vi "SyntaxToken.vi"(8 "error in":errorcluster, 9 "Error Index In":i32, 10 "Funcion Analizada":string, 11 "Logical Parsed Expression":T1) -> (0 "error out":errorcluster, 1 "Error Index Out":i32, 2 "Token":string[](array[string]), 3 "Logical Parsed Expression Out":T1)   [LabVIEW 2014]
uses:
  TypeDefs/LogicParsedExpression.ctl
  <vilib>/regexp/Match Regular Expression.xnode
  SeqLoop.lvlib
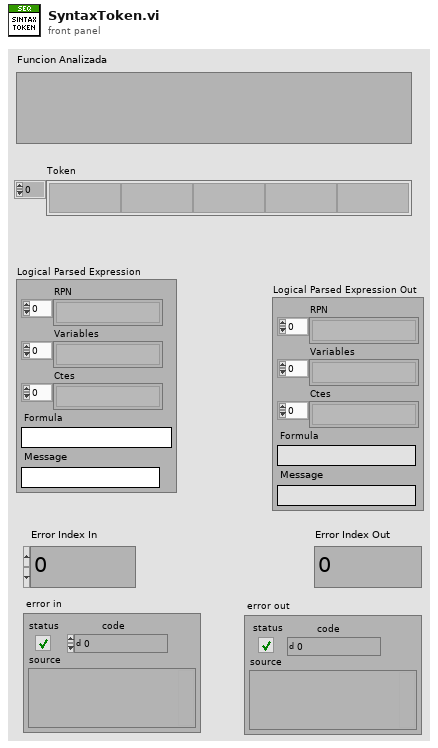
[diagram p1: front panel]
types:
  T1 = typedef "SeqLoop.lvlib/LogicParsedExpression.ctl" = cluster{"RPN ":string[], "Variables":string[], "Ctes":string[], "Formula":string, "Message":string}
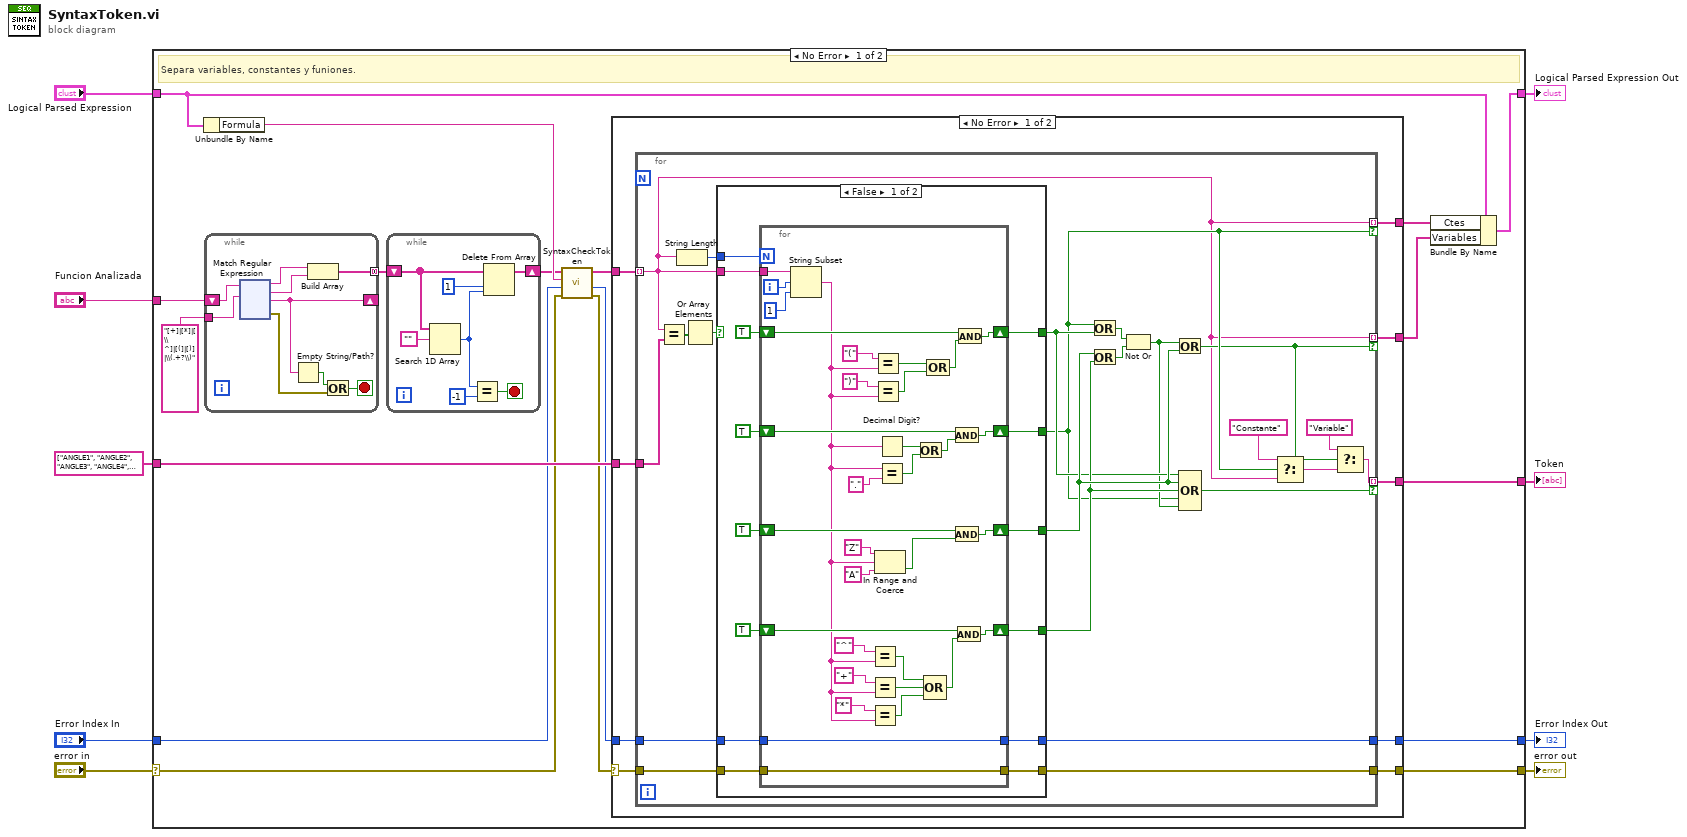
[diagram p0: block diagram]
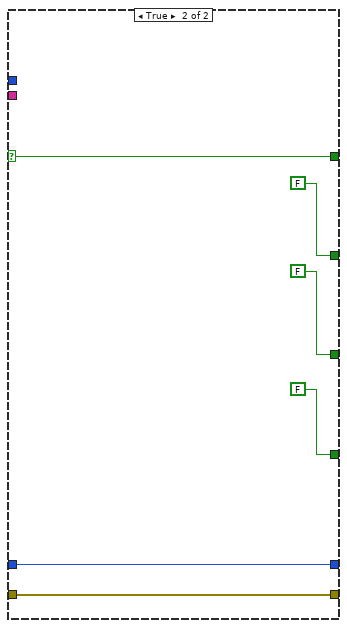
[diagram p2: hidden frame]
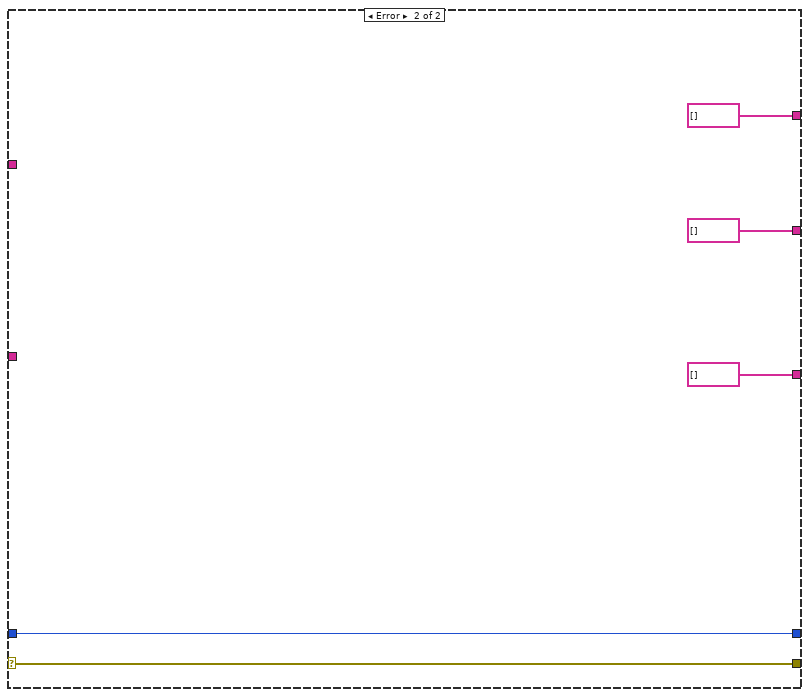
[diagram p3: hidden frame]
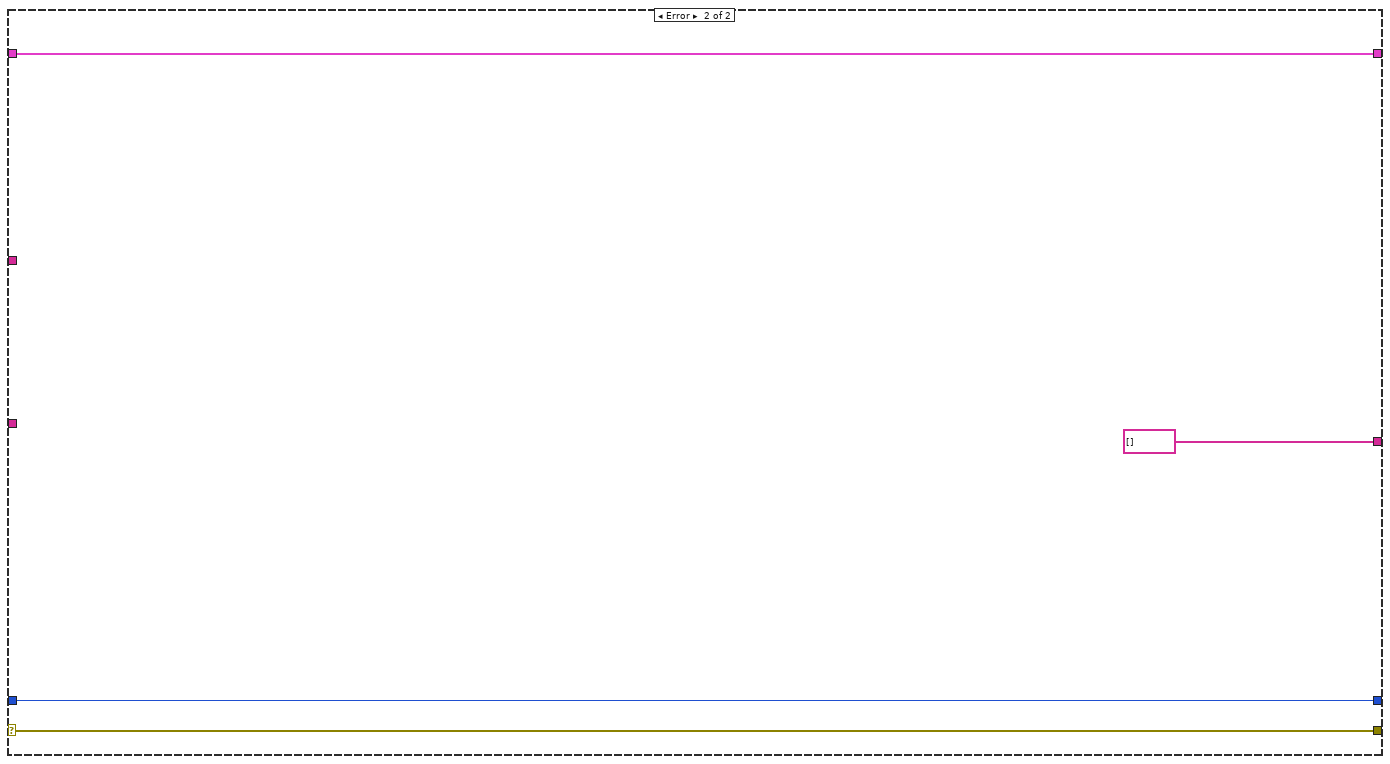
[diagram p4: hidden frame]
diagram:
  n1 = case shown="No Error" "error in" {
    selector: "error in" -> [w13 w250]
    tunnel: [w23 w250] -> w8
    tunnel: [w24 w249] -> w2
    tunnel: "Logical Parsed Expression" -> [w20 w249]
    tunnel: string[] ["ANGLE1", "ANGLE2", "ANGLE3", "ANGLE4", "ANGLE5", "NO", "W"] ("Funciones") -> [w22 _]
    tunnel: [w21 string[] []] -> w7
    tunnel: "Funcion Analizada" -> [w19 _]
    tunnel: "Error Index In" -> [w12 w247]
    tunnel: [w18 w247] -> w4
    frame No Error {
      # "Separa variables, constantes y funiones."
      n2 = Unbundle By Name(w20) -> ("Formula"=w11:string)
      n3 = while {
        tunnel: "[+]|[*]|[\\^]|[(]|[)]|\\(.+?\\)" ("regular expression") -> [w131]
        shift-right: [w130] -> _
        shift-left: w19 -> [w132]
        tunnel: [w129] -> w26 mode=concatenating
        stop <- w125 stop-if-true
        n4 = xnode "Match Regular Expression"("input string"=w132, "regular expression"=w131) -> ("before match"=w128:string, "whole match"=w127:string, "after match"=w130:string, "error out"=w124:errorcluster)  [unwired: 4 in, 1 out]
        n5 = Empty String/Path?(string/path=w130) -> (empty?=w126:bool)
        n6 = Build Array(w128, w127) -> (w129:string[])
        n7 = Or(x=w126, y=w124) -> (x .or. y?=w125:bool)
      }
      n8 = while {
        shift-right: [w117] -> w10
        shift-left: w26 -> [w121]
        stop <- w120 stop-if-true
        n9 = Search 1D Array(1D array=w121, element="") -> (index of element=w119:i32)  [unwired: 1 in]
        n10 = Equal?(x=w119, y=-1) -> (x = y?=w120:bool)
        n11 = Delete From Array(array=w121, length=1, index=w119) -> (array with subset deleted=w117:string[])  [unwired: 1 out]
      }
      n12 = call "SyntaxCheckToken.vi"("error in"=w13, "Error Index In"=w12, "Funcion"=w11, "SyntaxChek In"=w10) -> ("error out"=w15:errorcluster, "Error Index Out"=w16:i32, "SyntaxChek Out"=w14:string[])  [unwired: 5 in]
      n13 = case shown="No Error" w15 {
        selector: w15 -> [w31 w116]
        tunnel: [w36 string[] []] -> w25
        tunnel: [w35 w116] -> w23
        tunnel: w22 -> [w34 _]
        tunnel: [w33 string[] []] -> w21
        tunnel: w14 -> [w32 _]
        tunnel: w16 -> [w30 w113]
        tunnel: [w29 w113] -> w18
        tunnel: [w28 string[] []] -> w17
        frame No Error {
          n14 = for {
            tunnel: w32 -> [w37] mode=indexing
            tunnel: [w37] -> w28 mode=indexing if=w45
            tunnel: [w37] -> w36 mode=indexing if=w43
            tunnel: [w40] -> w33 mode=indexing if=w55
            tunnel: w34 -> [w46]
            tunnel: w31 -> [w47]
            tunnel: [w48] -> w35
            tunnel: w30 -> [w39]
            tunnel: [w38] -> w29
            n15 = Equal?(x=w37, y=w46) -> (x = y?=w57:bool[])
            n16 = String Length(string=w37) -> (length=w58:i32)
            n17 = Or Array Elements(Boolean array=w57) -> (logical OR=w56:bool)
            n18 = case shown="False" w56 {
              selector: w56 -> [_ w111]
              tunnel: w58 -> [w72 _]
              tunnel: w37 -> [w68 _]
              tunnel: [w66 w111] -> w50
              tunnel: [w65 FALSE ("digit?")] -> w51
              tunnel: [w63 FALSE ("digit?")] -> w52
              tunnel: [w64 FALSE ("digit?")] -> w45
              tunnel: [w62 w107] -> w48
              tunnel: w47 -> [w61 w107]
              tunnel: w39 -> [w60 w106]
              tunnel: [w59 w106] -> w38
              frame False {
                n19 = for {
                  N: w72 -> [_]
                  tunnel: w68 -> [w103]
                  shift-right: [w99] -> w64
                  shift-left: TRUE ("digit?") -> [w100]
                  shift-right: [w96] -> w63
                  shift-left: TRUE ("digit?") -> [w98]
                  shift-right: [w89] -> w65
                  shift-left: TRUE ("digit?") -> [w91]
                  shift-right: [w82] -> w66
                  shift-left: TRUE ("digit?") -> [w83]
                  tunnel: [w74] -> w62
                  tunnel: w61 -> [w74]
                  tunnel: w60 -> [w73]
                  tunnel: [w73] -> w59
                  i -> [w104]
                  n20 = String Subset(string=w103, offset (0)=w104, length (rest)=1 ("length (rest)")) -> (substring=w78:string)
                  n21 = Equal?(x="^" ("y"), y=w78) -> (x = y?=w80:bool)
                  n22 = Equal?(x="+" ("upper limit"), y=w78) -> (x = y?=w93:bool)
                  n23 = Equal?(x="*" ("upper limit"), y=w78) -> (x = y?=w92:bool)
                  n24 = Equal?(x="(" ("upper limit"), y=w78) -> (x = y?=w86:bool)
                  n25 = Equal?(x=")" ("upper limit"), y=w78) -> (x = y?=w87:bool)
                  n26 = In Range and Coerce(upper limit="Z", x=w78, lower limit="A" ("upper limit")) -> (In Range?=w97:bool)  [unwired: 1 out]
                  n27 = Decimal Digit?(1:w78) -> (0:w76:bool)
                  n28 = Equal?(x=w78, y=".") -> (x = y?=w75:bool)
                  n29 = Or(x=w76, y=w75) -> (x .or. y?=w77:bool)
                  n30 = Compound Arithmetic op=OR(w80, w93, w92) -> (w90:bool)
                  n31 = Compound Arithmetic op=OR(w86, w87) -> (w88:bool)
                  n32 = And(x=w100, y=w77) -> (x .and. y?=w99:bool)
                  n33 = And(x=w98, y=w97) -> (x .and. y?=w96:bool)
                  n34 = And(x=w91, y=w90) -> (x .and. y?=w89:bool)
                  n35 = And(x=w83, y=w88) -> (x .and. y?=w82:bool)
                }
              }
              frame True {
              }
            }
            n36 = Or(x=w45, y=w50) -> (x .or. y?=w54:bool)
            n37 = Or(x=w52, y=w51) -> (x .or. y?=w53:bool)
            n38 = Not Or(1:w53, 2:w54) -> (0:w49:bool)
            n39 = Or(x=w49, y=w52) -> (x .or. y?=w43:bool)
            n40 = Compound Arithmetic op=OR(w50, w52, w51, w45, w49) -> (w55:bool)
            n41 = Select(t="Constante" ("y"), s=w45, f=w37) -> (s? t:f=w41:string)
            n42 = Select(t="Variable" ("y"), s=w43, f=w41) -> (s? t:f=w40:string)
          }
        }
        frame Error {
        }
      }
      n43 = Bundle By Name(cluster=w20, "Ctes"=w17, "Variables"=w25) -> (w24:T1)
    }
    frame Error {
    }
  }
  "error out" <- w8
  "Token" <- w7
  "Error Index Out" <- w4
  "Logical Parsed Expression Out" <- w2
